vi "UnpackData.vi"(7 "NumChannels":i32, 8 "error In":errorcluster, 10 "1D Data In":dbl[](array[numeric])=[1.0, 2.0, 3.0, 4.0, 5.0, 6.0, 7.0, 8.0, 9.0]) -> (0 "error Out":errorcluster, 2 "2D Data Out":dbl[][](array[numeric]))   [LabVIEW 2017]
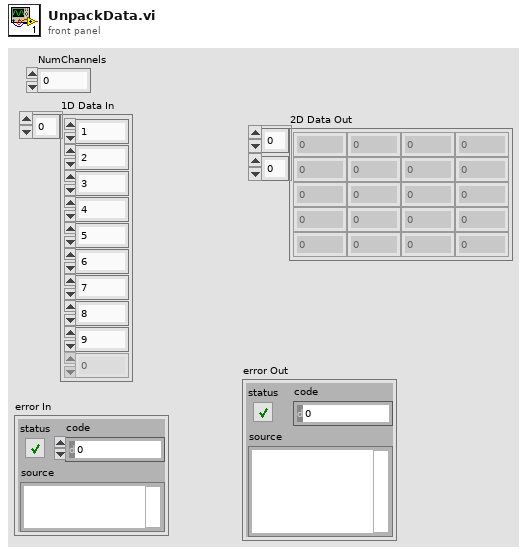
[diagram p1: front panel]
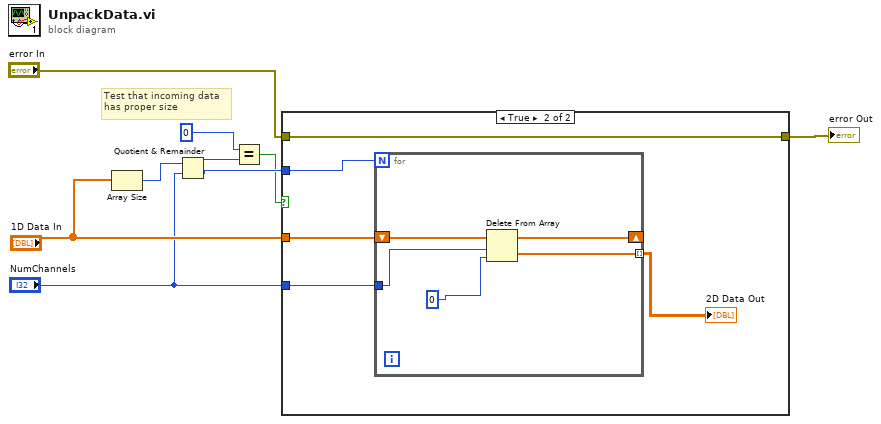
[diagram p0: block diagram]
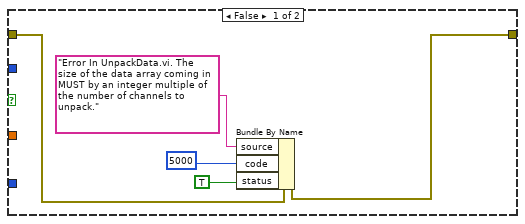
[diagram p2: hidden frame]
diagram:
  # "Test that incoming data\nhas proper size"
  n1 = Array Size(array="1D Data In") -> (size(s)=w8:i32)
  n2 = Quotient & Remainder(x=w8, y="NumChannels") -> (x-y*floor(x/y)=w2:i32, floor(x/y)=w3:i32)
  n3 = Equal?(x=0, y=w2) -> (x = y?=w1:bool)
  n4 = case shown="True" w1 {
    tunnel: "1D Data In" -> [_ w19]
    tunnel: "NumChannels" -> [_ w18]
    tunnel: "error In" -> [w13 w17]
    tunnel: [w14 w17] -> w4
    tunnel: w3 -> [_ w16]
    frame False {
      n5 = Bundle By Name(cluster=w13, "source"="Error In UnpackData.vi. The  size of the data array coming in MUST by an integer multiple of the number of channels to unpack.", "code"=5000, "status"=TRUE) -> (w14:errorcluster)
    }
    frame True {
      n6 = for {
        N: w16 -> [_]
        tunnel: w18 -> [w21]
        shift-right: [w23] -> _
        shift-left: w19 -> [w24]
        tunnel: [w20] -> w15 mode=indexing
        n7 = Delete From Array(array=w24, length=w21, index=0) -> (deleted portion=w20:dbl[], array with subset deleted=w23:dbl[])
      }
      "2D Data Out" <- w15
    }
  }
  "error Out" <- w4
